vi "AskForAPIKey.vi"(8 "error in (no error)":errorcluster) -> (0 "error out":errorcluster, 1 "String out":string, 2 "success?":bool caption="OK")   [LabVIEW 2019]
panel:
  in  "Cancel":bool
  in  "OK":bool caption="OK2"
  in  "String":string="Enter your ApiKey"
  # "Enter your ApiKey"
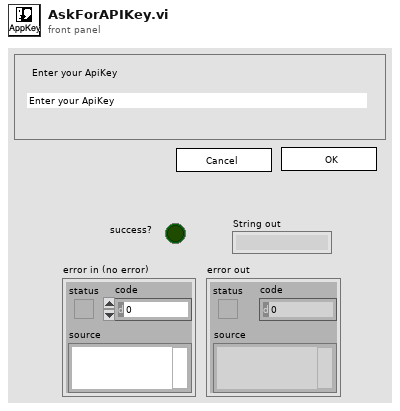
[diagram p1: front panel]
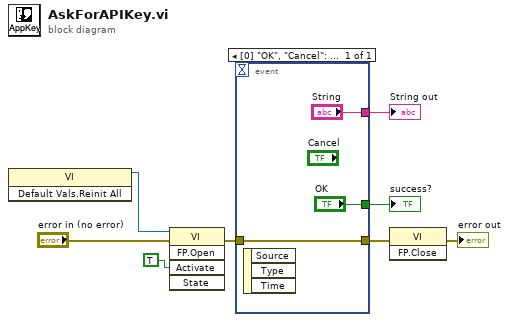
[diagram p0: block diagram]
diagram:
  n1 = invoke class="VI" method="Default Vals.Reinit All"() -> (reference out=w6:refnum<vi>)  [unwired: 3 in, 2 out]
  n2 = invoke class="VI" method="FP.Open"(reference=w6, error in="error in (no error)", "Activate"=TRUE ("Activate?")) -> (error out=w4:errorcluster)  [unwired: 2 in, 4 out]
  n3 = event shown="[0] \"OK\", \"Cancel\": Value Change;  Panel Close" {
    selector: _ -> [_]
    dyn-events: _ -> [_]
    timeout: _ -> [_]
    tunnel: ["OK"] -> w8
    tunnel: w4 -> [w10]
    tunnel: [w10] -> w3
    tunnel: ["String"] -> w1
    event "OK", "Cancel": Value Change; Panel Close {
      n4 = event-data() -> ()  [unwired: 1 in, 3 out]
    }
  }
  "success?" <- w8
  "String out" <- w1
  n5 = invoke class="VI" method="FP.Close"(error in=w3) -> (error out=→"error out":errorcluster)  [unwired: 2 in, 2 out]
